vi "ENV HAT.vi"() -> ()   [LabVIEW 2020]
uses:
  lv_waveforms_toolkit.lvlib
panel:
  out "pNak":i32
  out "rgbRx":u8[](array[numeric])
  out "Error Out":errorcluster
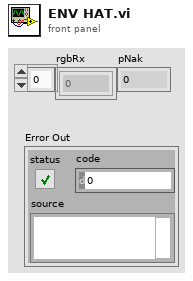
[diagram p1: front panel]
types:
  T1 = typedef "lv_waveforms_toolkit.lvlib/WFT Session.ctl" = cluster{"phdwf":i32, "Analog IO Configured":bool}
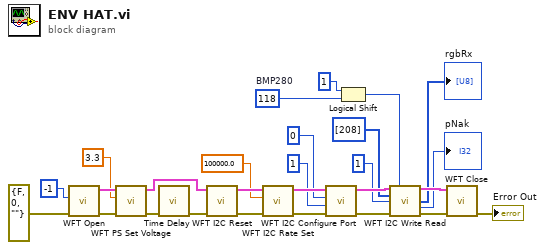
[diagram p0: block diagram]
diagram:
  w3 = u8 118  # BMP280
  n1 = call "WFT Open.vi"("Error In"=errorcluster {"status"=FALSE, "code"=0, "source"=""}, "idxDevice"=-1) -> ("Error Out"=w26:errorcluster, "WaveForms Session Out"=w27:T1)  [unwired: 7 in, 1 out]
  n2 = call "WFT PS Set Voltage.vi"("Error In"=w26, "Voltage"=3.3, "WaveForms Session In"=w27) -> ("Error Out"=w21:errorcluster, "WaveForms Session Out"=w16:T1)  [unwired: 7 in]
  n3 = call "Time Delay"("error in (no error)"=w21) -> ("error out"=w14:errorcluster)  [unwired: 10 in]
  n4 = call "WFT I2C Reset.vi"("Error In"=w14, "WaveForms Session In"=w16) -> ("Error Out"=w13:errorcluster, "WaveForms Session Out"=w15:T1)  [unwired: 7 in, 1 out]
  n5 = call "WFT I2C Rate Set.vi"("Error In"=w13, "hz"=100000.0, "WaveForms Session In"=w15) -> ("Error Out"=w19:errorcluster, "WaveForms Session Out"=w20:T1)  [unwired: 6 in, 1 out]
  n6 = call "WFT I2C Configure Port.vi"("Error In"=w19, "SDA idxChannel"=1, "SCL idxChannel"=0, "WaveForms Session In"=w20) -> ("Error Out"=w10:errorcluster, "WaveForms Session Out"=w11:T1)  [unwired: 4 in, 2 out]
  n7 = Logical Shift(y=i16 1, x=w3) -> (x << y=w1:u8)
  n8 = call "WFT I2C Write Read.vi"("WaveForms Session In"=w11, "adr8Bits"=w1, "rgbTx"=u8[] [208], "cRx"=1, "Error In"=w10) -> ("WaveForms Session Out"=w8:T1, "rgbRx"=→"rgbRx":u8[], "pNak"=→"pNak":i32, "Error Out"=w9:errorcluster)  [unwired: 6 in, 1 out]
  n9 = call "WFT Close.vi"("Error In"=w9, "WaveForms Session In"=w8) -> ("Error Out"=→"Error Out":errorcluster)  [unwired: 8 in, 1 out]
